vi "Mem_WaveformArray.vi"(8 "error in (no error)":errorcluster, 11 "dataInfo":T1) -> (0 "error out":errorcluster, 2 "Array":waveform(dbl)[](array[waveform]))   [LabVIEW 2019, in "Memory Data Access.lvlib"]
uses:
  Memory Data Access.lvlib
  Typedef/memoryDataBlock.ctl
  Global/Global.vi
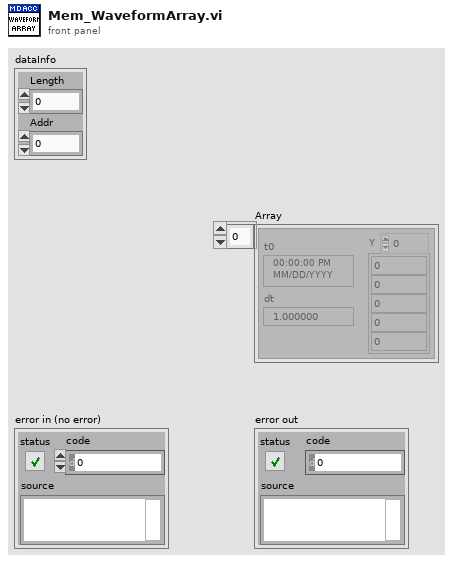
[diagram p1: front panel]
types:
  T1 = typedef "Memory Data Access.lvlib/memoryDataBlock.ctl" = cluster{"Length":u32, "Addr":u64}
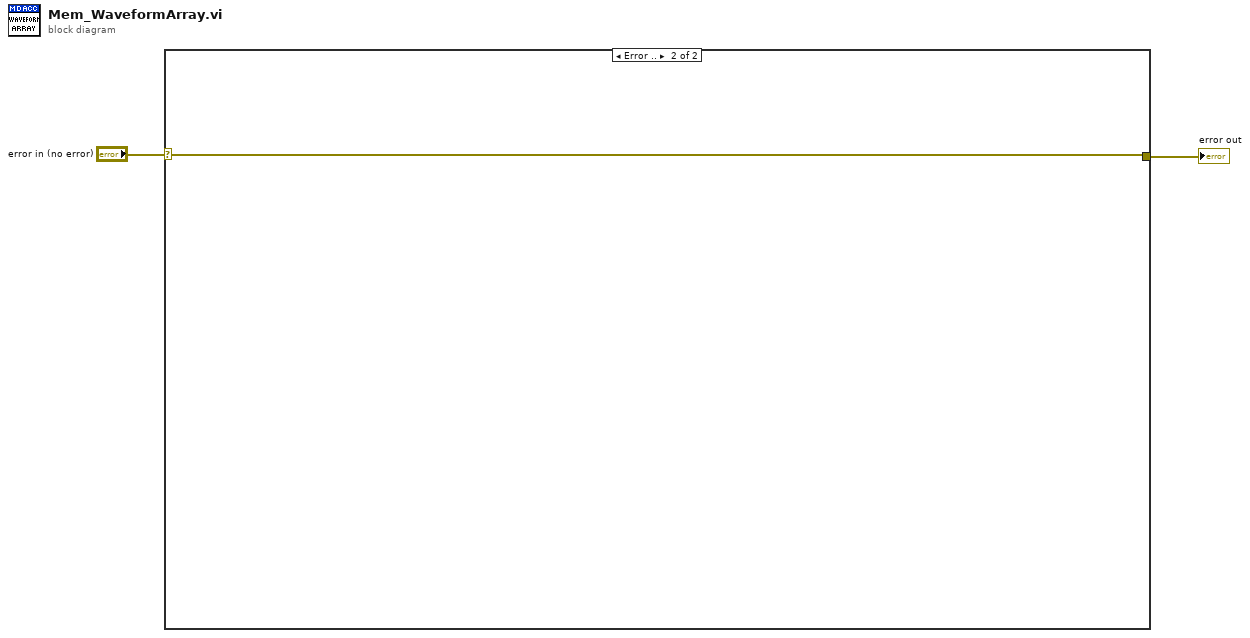
[diagram p0: block diagram]
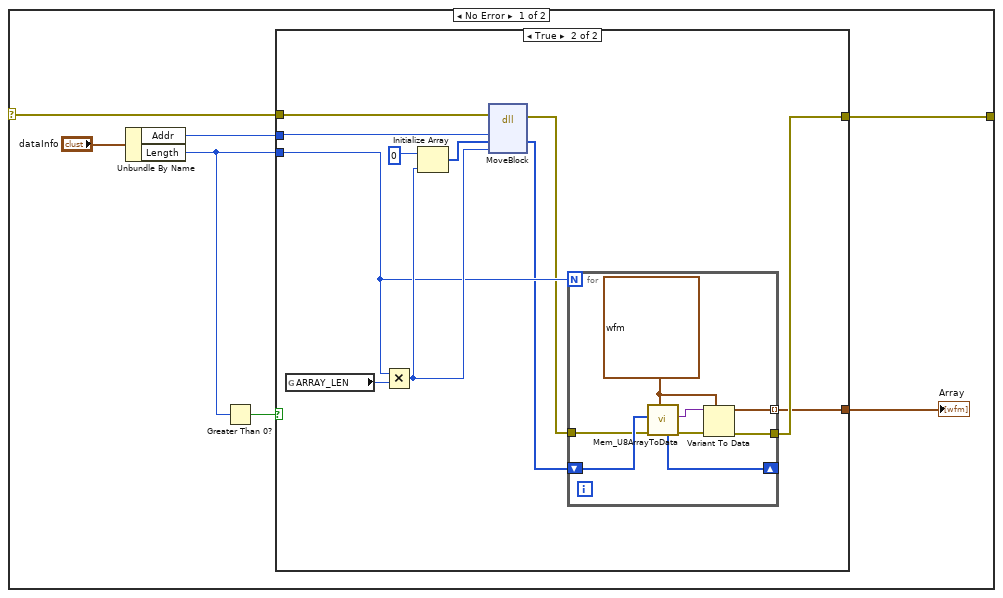
[diagram p2: hidden frame]
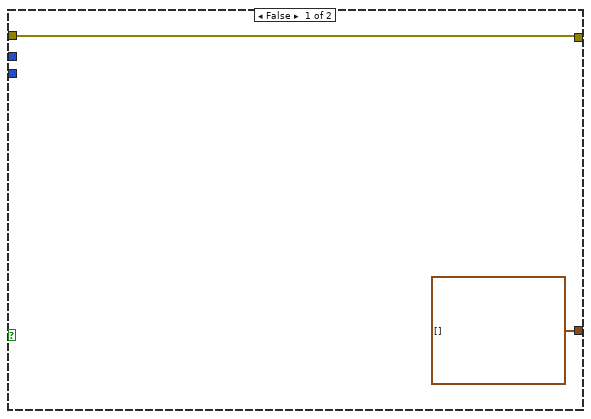
[diagram p3: hidden frame]
diagram:
  n1 = case shown="Error .." "error in (no error)" {
    selector: "error in (no error)" -> [w9 w31]
    tunnel: [w8 w31] -> w1
    frame No Error {
      n2 = Unbundle By Name("dataInfo") -> ("Addr"=w5:u64, "Length"=w4:u32)
      n3 = Greater Than 0?(x=w4) -> (x > 0?=w7:bool)
      n4 = case shown="True" w7 {
        tunnel: w9 -> [w11 w22]
        tunnel: [w11 w13] -> w8
        tunnel: w5 -> [_ w19]
        tunnel: w4 -> [_ w16]
        tunnel: [waveform(dbl)[] [] w12] -> w3
        frame False {
        }
        frame True {
          n5 = global read "Global.vi" "ARRAY_LEN"() -> (w18:u32)
          n6 = Multiply(x=w16, y=w18) -> (x*y=w17:u32)
          n7 = Initialize Array(u8 0, w17) -> (w20:u8[])
          n8 = dll-call lib="LabVIEW" fn="MoveBlock"(error in=w22, "Address"=w19, "Destination"=w20, "Size"=w17) -> (error out=w14:errorcluster, "Destination"=w15:u8[])  [unwired: 5 in, 1 out]
          n9 = for {
            N: w16 -> [_]
            shift-right: [w29] -> _
            shift-left: w15 -> [w30]
            tunnel: [w25] -> w12 mode=indexing
            tunnel: [w24] -> w13
            tunnel: w14 -> [w23]
            w26 = waveform(dbl) {"t0"=timestamp(0 s since 1904-01-01), "dt"=1.0, "Y"=[]} ("Waveform")
            n10 = call "Mem_U8ArrayToData.vi"("Type"=w26, "error in (no error)"=w23, "ByteArray"=w30) -> ("error out"=w28:errorcluster, "data"=w27:variant, "ByteArray Left"=w29:u8[])  [unwired: 5 in, 1 out]
            n11 = Variant To Data(error in=w28, type=w26, Variant=w27) -> (data=w25:waveform(dbl), error out=w24:errorcluster)
          }
        }
      }
      "Array" <- w3
    }
    frame Error {
    }
  }
  "error out" <- w1
